vi "Magnet test.vi"() -> ()   [LabVIEW 2012]
panel:
  in  "B_z":dbl
  in  "B_y":dbl
  in  "B_x":dbl
  in  "stop":bool
  out "X (uT)":dbl
  out "Y (uT)":dbl
  out "Z (uT)":dbl
  out "Waveform Chart":dbl(graph)
  out "Waveform Chart 2":dbl(graph)
  out "Waveform Chart 3":dbl(graph)
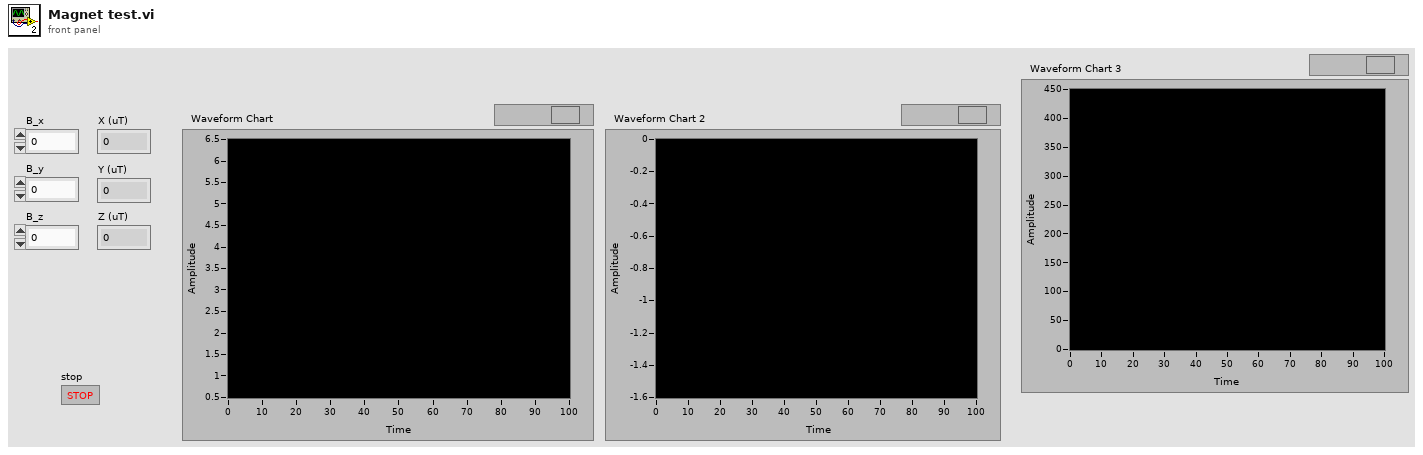
[diagram p1: front panel]
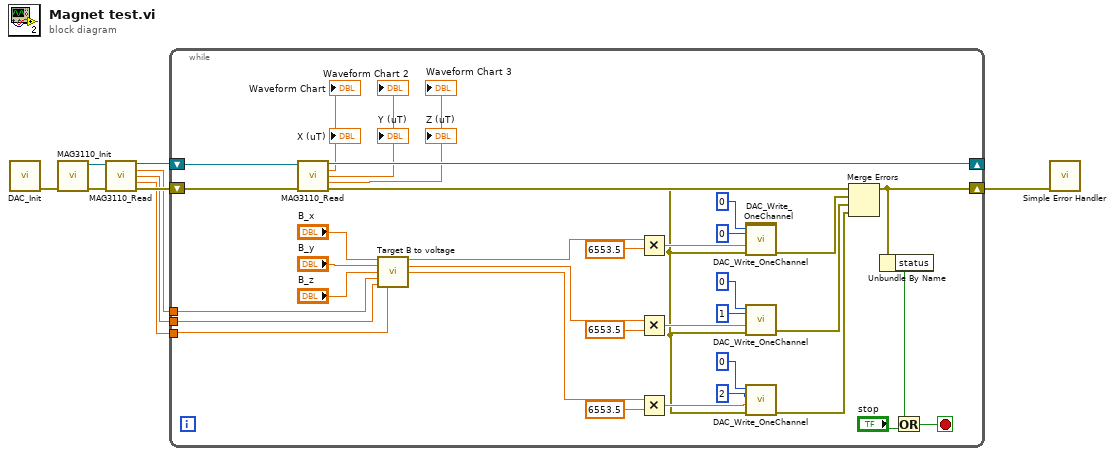
[diagram p0: block diagram]
diagram:
  n1 = call "DAC_Init.vi"() -> ("error out"=w9:errorcluster)  [unwired: 11 in]
  n2 = call "MAG3110_Init.vi"("error in (no error)"=w9) -> ("VISA resource name out"=w7:refnum<visa-resource-name>, "error out"=w5:errorcluster)  [unwired: 8 in]
  n3 = call "MAG3110_Read.vi"("VISA resource name"=w7, "error in (no error)"=w5) -> ("VISA resource name out"=w6:refnum<visa-resource-name>, "X (uT)"=w3:dbl, "Y (uT)"=w2:dbl, "Z (uT)"=w1:dbl, "error out"=w4:errorcluster)  [unwired: 9 in]
  n4 = while {
    shift-right: [w43] -> _
    shift-left: w6 -> [w44]
    shift-right: [w23] -> w8
    shift-left: w4 -> [w28]
    tunnel: w3 -> [w12]
    tunnel: w2 -> [w11]
    tunnel: w1 -> [w10]
    stop <- w24 stop-if-true
    n5 = call "MAG3110_Read.vi"("VISA resource name"=w44, "error in (no error)"=w28) -> ("VISA resource name out"=w43:refnum<visa-resource-name>, "X (uT)"=→"X (uT)" →"Waveform Chart":dbl, "Y (uT)"=→"Y (uT)" →"Waveform Chart 2":dbl, "Z (uT)"=→"Z (uT)" →"Waveform Chart 3":dbl, "error out"=w42:errorcluster)  [unwired: 9 in]
    n6 = call "Target B to voltage.vi"("B_x"="B_x", "B_y"="B_y", "B_z"="B_z", "Earth B_x"=w12, "Earth B_y"=w11, "Earth B_z"=w10) -> ("element"=w15:dbl, "element 2"=w14:dbl, "element 3"=w13:dbl)  [unwired: 7 in]
    n7 = Multiply(x=w15, y=6553.5) -> (x*y=w38:dbl)
    n8 = Multiply(x=w14, y=6553.5) -> (x*y=w30:dbl)
    n9 = Multiply(x=w13, y=6553.5) -> (x*y=w29:dbl)
    n10 = call "DAC_Write_OneChannel.vi"() -> ()  [unwired: 10 in, 2 out]
    n11 = call "DAC_Write_OneChannel.vi"("error in (no error)"=w28, "Value"=w38, "Channel"=u16 0, "DeviceIndex"=u64 0) -> ("error out"=w41:errorcluster)  [unwired: 6 in, 1 out]
    n12 = call "DAC_Write_OneChannel.vi"("error in (no error)"=w28, "Value"=w30, "Channel"=u16 1, "DeviceIndex"=u64 0) -> ("error out"=w27:errorcluster)  [unwired: 6 in, 1 out]
    n13 = call "DAC_Write_OneChannel.vi"("error in (no error)"=w28, "Value"=w29, "Channel"=u16 2, "DeviceIndex"=u64 0) -> ("error out"=w26:errorcluster)  [unwired: 6 in, 1 out]
    n14 = Merge Errors(w42, w41, w27, w26) -> (w23:errorcluster)
    n15 = Unbundle By Name(w23) -> ("status"=w22:bool)
    n16 = Or(x=w22, y="stop") -> (x .or. y?=w24:bool)
  }
  n17 = call <vilib>:"Simple Error Handler.vi"("error in (no error)"=w8) -> ()  [unwired: 4 in, 5 out]
